vi "MPU_Stick_Read_Serial_Port_Emulator.vi"() -> ()   [LabVIEW 2017]
panel:
  out "Read Serial Port Emulator":bool
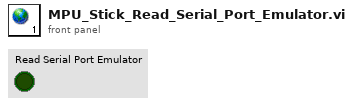
[diagram p1: front panel]
diagram:
